vi "Save.vi"(8 "error in (no error)":errorcluster, 11 "App Config Data In":T1) -> (0 "error out":errorcluster, 3 "App Config Data Out":T1)   [LabVIEW 2015, in "App Config.lvlib"]
uses:
  App Config.lvlib
  App Config Data.ctl
  <vilib>/Utility/xml.llb/Write to XML File(string).vi
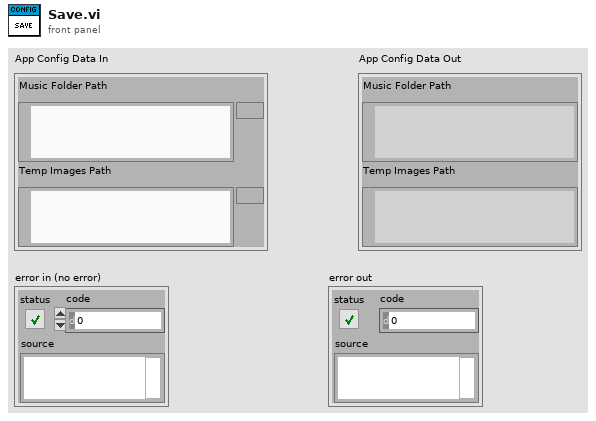
[diagram p1: front panel]
types:
  T1 = typedef "App Config.lvlib/App Config Data.ctl" = cluster{"Music Folder Path":path, "Temp Images Path":path}
  T2 = enum16{"open", "replace", "create", "open or create", "replace or create", "replace or create with confirmation"}
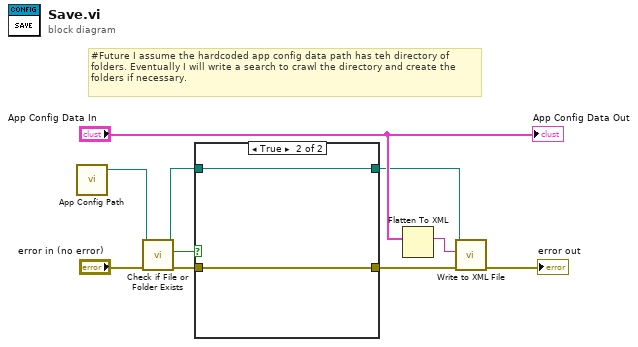
[diagram p0: block diagram]
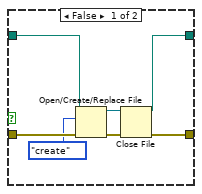
[diagram p2: hidden frame]
diagram:
  # "#Future I assume the hardcoded app config data path has teh directory of folders. Eventually I will write a search to crawl the directory and create the folders if necessary."
  n1 = call "App Config Path.vi"() -> ("App Config Path"=w9:path)  [unwired: 5 in]
  n2 = call <vilib>:"Check if File or Folder Exists.vi"("error in (no error)"="error in (no error)", "path"=w9) -> ("error out"=w5:errorcluster, "file or folder exists?"=w4:bool, "dup path"=w3:path)  [unwired: 7 in]
  n3 = case shown="True" w4 {
    tunnel: w5 -> [w17 w18]
    tunnel: w3 -> [w13 w19]
    tunnel: [w12 w19] -> w2
    tunnel: [w11 w18] -> w1
    frame False {
      n4 = Open/Create/Replace File(file path (use dialog)=w13, error in=w17, operation (0:open)=T2."create") -> (refnum out=w14:refnum<file>, error out=w15:errorcluster)  [unwired: 3 in, 1 out]
      n5 = Close File(refnum=w14, error in=w15) -> (path=w12:path, error out=w11:errorcluster)
    }
    frame True {
    }
  }
  n6 = Flatten To XML(anything="App Config Data In") -> (xml string=w7:string)
  n7 = call-poly <vilib>:"Write to XML File.vi"("error in (no error)"=w1, "XML Input"=w7, "XML File Path"=w2) -> ("error out"=→"error out":errorcluster)  [unwired: 6 in, 2 out]
  "App Config Data Out" <- "App Config Data In"
